vi "SD Write Position Names.vi"() -> ()   [LabVIEW 2020]
uses:
  SD Type Defs/SD Position Names.ctl
panel:
  in  "Cancel":bool
  in  "Save":bool
  in  "Dichroic Names":string[](array[string])
  in  "Filter Names":string[](array[string])
  in  "Disk Pattern Names":string[](array[string])
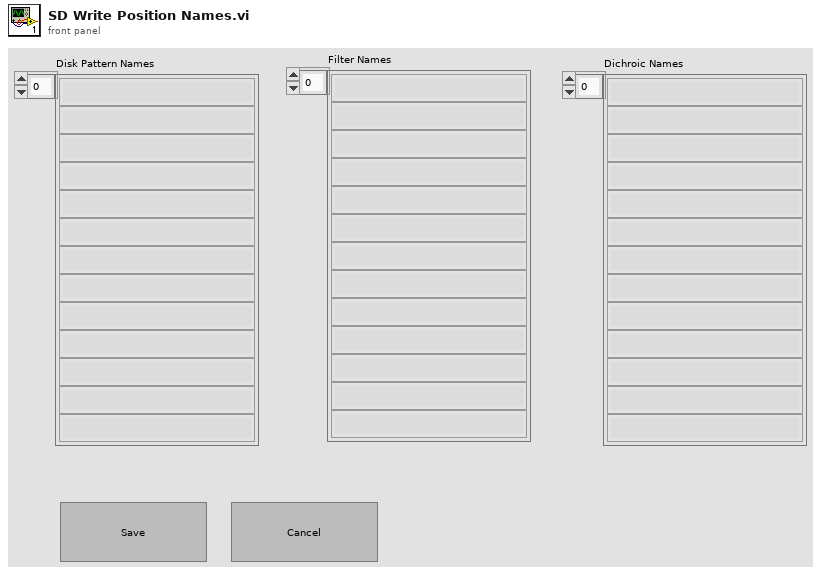
[diagram p1: front panel]
types:
  T1 = typedef "SD Position Names.ctl" = cluster{"Disk Patterns":string[], "Filters":string[], "Dichroics":string[]}
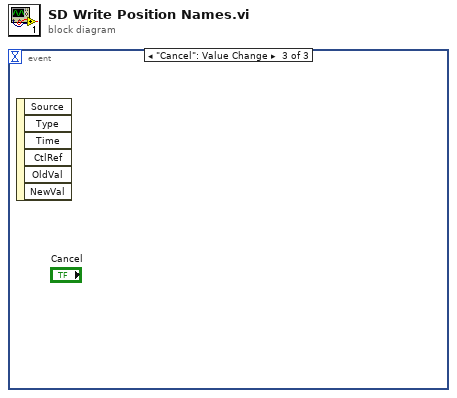
[diagram p0: block diagram]
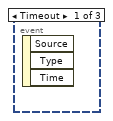
[diagram p2: hidden frame]
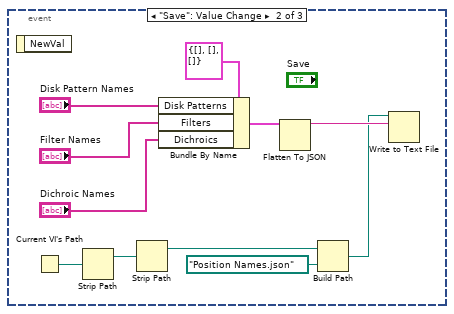
[diagram p3: hidden frame]
diagram:
  n1 = event shown="[2] \"Cancel\": Value Change" {
    selector: _ -> [_ _ _]
    dyn-events: _ -> [_ _ _]
    timeout: _ -> [_ _ _]
    event Timeout {
      n2 = event-data() -> ()  [unwired: 1 in, 3 out]
    }
    event "Save": Value Change {
      n3 = event-data() -> ()  [unwired: 1 in, 1 out]
      n4 = Current VI's Path() -> (path=w6:path)
      n5 = Strip Path(path=w6) -> (stripped path=w4:path)  [unwired: 1 out]
      n6 = Strip Path(path=w4) -> (stripped path=w3:path)  [unwired: 1 out]
      n7 = Bundle By Name(cluster=T1 {"Disk Patterns"=[], "Filters"=[], "Dichroics"=[]} ("SD Names"), "Disk Patterns"="Disk Pattern Names", "Filters"="Filter Names", "Dichroics"="Dichroic Names") -> (w7:T1)
      n8 = Flatten To JSON(anything=w7) -> (JSON string=w2:string)  [unwired: 2 in, 1 out]
      n9 = Build Path(base path=w3, name or relative path=path "Position Names.json") -> (appended path=w1:path)
      n10 = Write to Text File(file (use dialog)=w1, text=w2) -> ()  [unwired: 2 in, 3 out]
    }
    event "Cancel": Value Change {
      n11 = event-data() -> ()  [unwired: 1 in, 6 out]
    }
  }
